vi "Read Lines From File - no popup.vi"(2 "convert eol? (no:F)":bool, 3 "file path (dialog if empty)":path, 4 "number of lines (all:-1)":i32=-1, 8 "start of read offset (chars.:0)":i32, 9 "[max characters per line]  (no limit:0)":i32) -> (0 "new file path (Not A Path if cancelled)":path, 1 "line string":string, 5 "mark after read (chars.)":i32, 6 "EOF?":bool)   [LabVIEW 2013]
doc: "LabVIEW no longer supports this VI. Use the Read Text function instead. Reads a specified number of lines from a byte stream file beginning at a specified character offset. The VI opens the file before reading from it and closes it afterwards."
uses:
  <vilib>/Utility/error.llb/DialogType.ctl
panel:
  out "error out":errorcluster
  in  "prompt":string="Choose file to read."
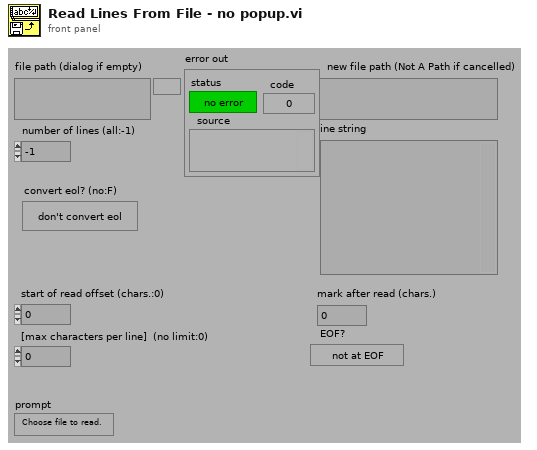
[diagram p1: front panel]
types:
  T1 = typedef "DialogType.ctl" = u16
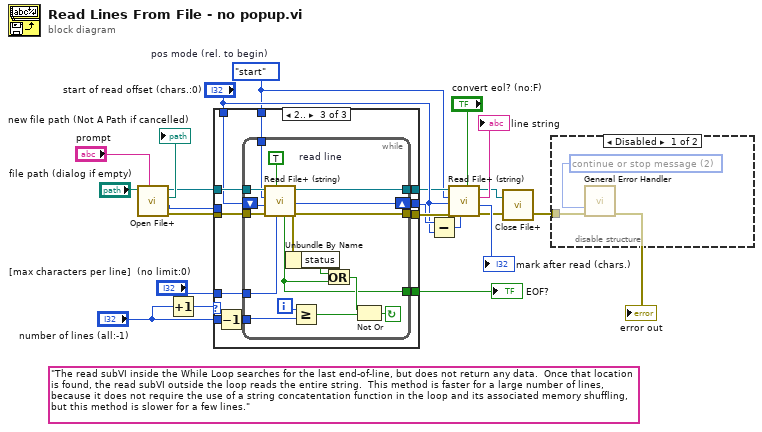
[diagram p0: block diagram]
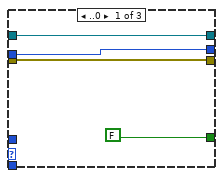
[diagram p3: hidden frame]
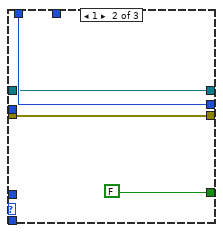
[diagram p4: hidden frame]
diagram:
  w10 = enum16{"start", "end", "current"}."start"  # pos mode (rel. to begin)
  (unwired) "The read subVI inside the While Loop searches for the last end-of-line, but does not return any data.  Once that location is found, the read subVI outside the loop reads the entire string.  This method is faster for a large number of lines, because it does not require the use of a string concatentation function in the loop and its associated memory shuffling, but this method is slower for a few lines."
  n1 = call <vilib>:"Open File+.vi"("prompt"="prompt", "file path (\" \")"="file path (dialog if empty)") -> ("error out"=w9:errorcluster, "file size (bytes)"=w8:i32, "file path"=→"new file path (Not A Path if cancelled)":path, "refnum"=w6:refnum<file>)  [unwired: 6 in]
  n2 = Increment(x="number of lines (all:-1)") -> (x+1=w16:i32)
  n3 = case shown="2.." w16 {
    tunnel: [w26 w29 w41] -> w18
    tunnel: [w25 w30 w40] -> w17
    tunnel: "number of lines (all:-1)" -> [_ _ w39]
    tunnel: "[max characters per line]  (no limit:0)" -> [_ _ w38]
    tunnel: w9 -> [w26 w29 w37]
    tunnel: w6 -> [w24 w28 w36]
    tunnel: "start of read offset (chars.:0)" -> [_ w30 w35]
    tunnel: w10 -> [_ _ w34]
    tunnel: w8 -> [w25 _ _]
    tunnel: [w24 w28 w33] -> w13
    tunnel: [FALSE FALSE w32] -> w12
    frame ..0 {
    }
    frame 1 {
    }
    frame 2.. {
      n4 = Decrement(x=w39) -> (x-1=w31:i32)
      n5 = while {
        tunnel: [w43] -> w32
        tunnel: w34 -> [w48]
        tunnel: w37 -> [w50]
        tunnel: w38 -> [w51]
        tunnel: [w46] -> w41
        tunnel: w36 -> [w53]
        tunnel: [w54] -> w33
        tunnel: w31 -> [w42]
        shift-left: w35 -> [w55]
        shift-right: [w57] -> w40
        i -> [w56]
        stop <- w49 continue-if-true
        w45 = TRUE  # read line
        n6 = call <vilib>:"Read File+ (string).vi"("count"=w51, "line mode (characters:F)"=w45, "error in (no error)"=w50, "pos offset (bytes:0)"=w55, "pos mode (rel. to current:2)"=w48, "refnum"=w53) -> ("error out"=w46:errorcluster, "mark after read (bytes)"=w57:i32, "dup refnum"=w54:refnum<file>, "EOF?"=w43:bool)  [unwired: 1 in, 1 out]
        n7 = Unbundle By Name(w46) -> ("status"=w44:bool)
        n8 = Greater Or Equal?(x=w56, y=w42) -> (x >= y?=w52:bool)
        n9 = Or(x=w44, y=w43) -> (x .or. y?=w47:bool)
        n10 = Not Or(1:w52, 2:w47) -> (0:w49:bool)
      }
    }
  }
  "EOF?" <- w12
  n11 = Subtract(x=w17, y="start of read offset (chars.:0)") -> (x-y=w22:i32)
  n12 = call <vilib>:"Read File+ (string).vi"("convert eol? (no:F)"="convert eol? (no:F)", "count"=w22, "error in (no error)"=w18, "pos offset (bytes:0)"="start of read offset (chars.:0)", "pos mode (rel. to current:2)"=w10, "refnum"=w13) -> ("error out"=w3:errorcluster, "mark after read (bytes)"=→"mark after read (chars.)":i32, "string"=→"line string":string, "dup refnum"=w1:refnum<file>)  [unwired: 1 in, 1 out]
  n13 = call <vilib>:"Close File+.vi"("error in (no error)"=w3, "refnum"=w1) -> ("error out"=w2:errorcluster)  [unwired: 3 in, 2 out]
  "error out" <- w2
  n14 = disable-structure shown="Disabled" {
    disable-tunnel: w2 -> [w58 _]
    frame Disabled {
      w59 = T1 2 items=["no dialog", "OK message", "continue or stop message", "OK message + warnings", "continue/stop + warnings"] ("type of dialog (OK msg:1)")
      n15 = call <vilib>:"General Error Handler.vi"("type of dialog (OK msg:1)"=w59, "error in (no error)"=w58) -> ()  [unwired: 9 in, 5 out]
    }
    frame Enabled {
    }
  }
